vi "Unflatten.vi"(8 "error in (no error)":errorcluster, 9 "timeout in":bool, 10 "Data in":T1[](array[typedef]), 11 "CIFFifoCAN in":refnum<class "CIF_NIChn_Fifo_Power.lvclass">) -> (0 "error out":errorcluster, 2 "Data out":T1[](array[typedef]), 3 "CIFFifoCAN out":refnum<class "CIF_NIChn_Fifo_Power.lvclass">, 4 "Header":T2)   [LabVIEW 2021, in "CIF_NIChn_Fifo_Power.lvclass"]
uses:
  CIF_NIChn_Fifo_Power.lvclass
  D:/dev/Packages/Channel_Manager/src/CIFChannels/CIFChannels.lvclass
  ChannelCommon/typedef/FIFO Header.ctl
  ChannelCommon/typedef/Datatype Waveform.ctl
  CIFChannels/CIFChannels.lvclass/CIFChannels.ctl
  CIF_NIChn_Fifo_Power.lvclass/CIF_NIChn_Fifo_Power.ctl
  CIFChannels/Accessors/Write FIFO Header.vi
  CIFChannels/Accessors/Write FIFO Timeout.vi
  ChannelCommon/Utilities/Unflatten Header.vi
  <vilib>/CIF Foundation/CIF Utilities/DataTypes/Unflatten I64.vi
  ChannelCommon/CIFFIFO/Flatten/Waveform Unflatten.vi/ce8ba92d-590f-4e46-8b1c-68dfd5c82777.vi
  ChannelCommon/CIFFIFO/Flatten/Waveform Unflatten.vi/8980f996-a542-42f1-9c98-910966e77ad2.vi
  <vilib>/CIF Foundation/CIF Utilities/DataTypes/Unflatten U64.vi
  ChannelCommon/Utilities/Add Error.vi
  ChannelCommon/CIFFIFO/Flatten/Waveform Unflatten.vi/ce8ba92d-590f-4e46-8b1c-68dfd5c82777.vi/c28b0ead-42ad-4072-80a2-aca7f2bd7ce3.vi
  ChannelCommon/CIFFIFO/Flatten/Waveform Unflatten.vi/8980f996-a542-42f1-9c98-910966e77ad2.vi/c28b0ead-42ad-4072-80a2-aca7f2bd7ce3.vi
  <vilib>/CIF Foundation/CIF Utilities/Errors/Append Error Location.vi
  ChannelCommon/ChannelCommon.lvlib
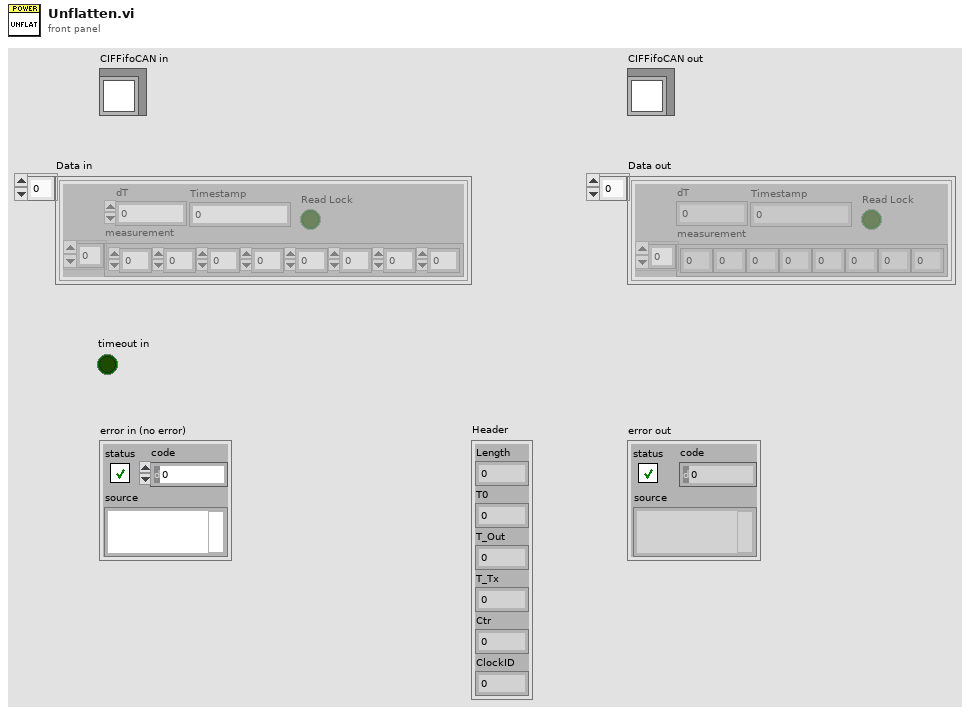
[diagram p1: front panel]
types:
  T1 = typedef "ChannelCommon.lvlib/Datatype Waveform.ctl" = cluster{"measurement":dbl[], "dT":dbl, "Timestamp":i64, "Read Lock":bool}
  T2 = typedef "ChannelCommon.lvlib/FIFO Header.ctl" = cluster{"Length":u64, "T0":i64, "T_Out":i64, "T_Tx":i64, "Ctr":u64, "ClockID":u8}
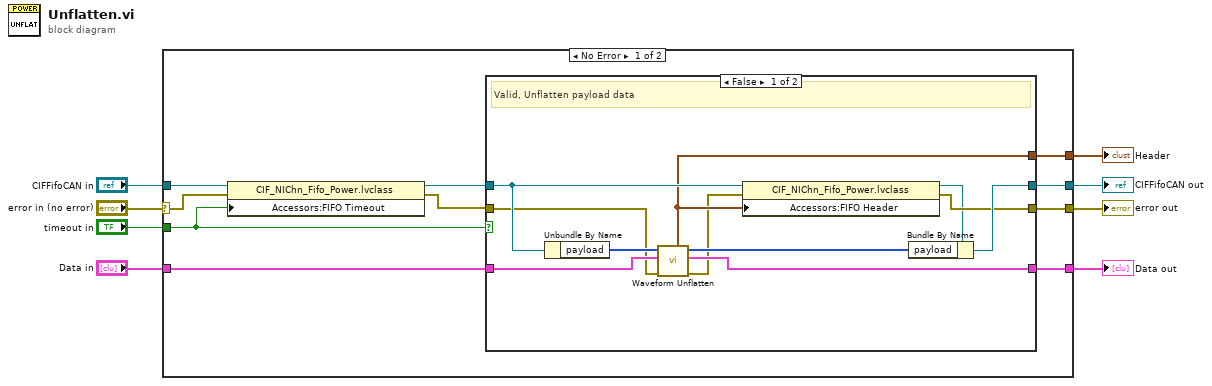
[diagram p0: block diagram]
diagram:
  n1 = case shown="No Error" "error in (no error)" {
    selector: "error in (no error)" -> [w12 w33]
    tunnel: [w15 w33] -> w7
    tunnel: [w16 w32] -> w5
    tunnel: "CIFFifoCAN in" -> [w13 w32]
    tunnel: "timeout in" -> [w11 _]
    tunnel: [w18 _] -> w2
    tunnel: [w17 _] -> w3
    tunnel: "Data in" -> [w14 _]
    frame No Error {
      n2 = property class="CIF_NIChn_Fifo_Power.lvclass"(reference=w13, error in=w12, "Accessors:FIFO Timeout"=w11) -> (reference out=w10:refnum<class "CIF_NIChn_Fifo_Power.lvclass">, error out=w9:errorcluster)
      n3 = case shown="False" w11 {
        tunnel: w9 -> [w19 w30]
        tunnel: w10 -> [w24 w31]
        tunnel: [w29 _] -> w18
        tunnel: [w23 _] -> w17
        tunnel: [w28 w31] -> w16
        tunnel: [w21 w30] -> w15
        tunnel: w14 -> [w27 _]
        frame False {
          # "Valid, Unflatten payload data"
          n4 = Unbundle By Name(w24) -> ("payload"=w25:u8[])
          n5 = call "Waveform Unflatten.vi"("error in (no error)"=w19, "Data in in"=w27, "Flatten Data in"=w25) -> ("error out"=w22:errorcluster, "Data out"=w29:T1[], "Flatten Data out"=w26:u8[], "Header out"=w23:T2)  [unwired: 5 in]
          n6 = property class="CIF_NIChn_Fifo_Power.lvclass"(reference=w24, error in=w22, "Accessors:FIFO Header"=w23) -> (reference out=w20:refnum<class "CIF_NIChn_Fifo_Power.lvclass">, error out=w21:errorcluster)
          n7 = Bundle By Name(cluster=w20, "payload"=w26) -> (w28:refnum<class "CIF_NIChn_Fifo_Power.lvclass">)
        }
        frame True {
          # "Timeout"
        }
      }
    }
    frame Error {
    }
  }
  "error out" <- w7
  "CIFFifoCAN out" <- w5
  "Header" <- w3
  "Data out" <- w2
